vi "ANDOR_GetSoftwareVersion.vi"(7 "error in (no error)":errorcluster) -> (18 "Software Versions":T1, 20 "eprom":u32, 21 "cofFile":u32, 22 "vxdRev":u32, 23 "vxdVer":u32, 24 "dllRev":u32, 25 "dllVer":u32, 26 "DLL error code":u32, 27 "error out":errorcluster)   [LabVIEW 2010]
doc: "This function returns the Software version information for the microprocessor code and the driver.\n\n<B>Parameters:</B>\neprom - EPROM version\ncofFile - COF file version\nvxdRev - Driver revision number\nvxdVer - Driver version number\ndllRev - DLL revision number\ndllVer - DLL version number\n\n<B>Error codes:</B>\nDRV_SUCCESS - Version information returned.\nDRV_NOT_INITIALIZED - System not initialized.\nDRV_ACQUIRING - Acquisition in progress.\nDRV_ERROR_ACK - Unable to communicate with card."
uses:
  Program Files/Andor SOLIS/atmcd32d.dll
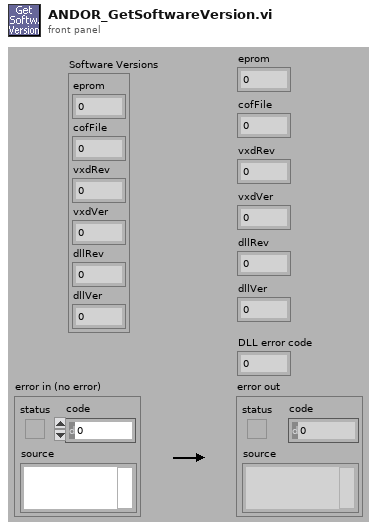
[diagram p1: front panel]
types:
  T1 = cluster{"eprom":u32, "cofFile":u32, "vxdRev":u32, "vxdVer":u32, "dllRev":u32, "dllVer":u32}
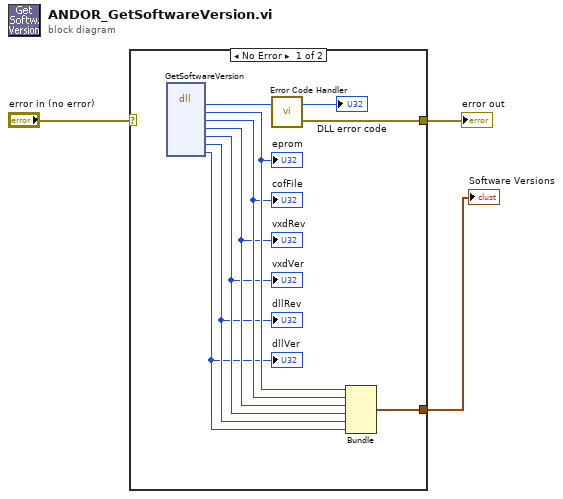
[diagram p0: block diagram]
diagram:
  n1 = case shown="No Error" "error in (no error)" {
    selector: "error in (no error)" -> [_ w14]
    tunnel: [w12 w14] -> w2
    tunnel: [w4 _] -> w1
    frame No Error {
      n2 = dll-call lib="C:/Program Files/Andor SOLIS/atmcd32d.dll" fn="GetSoftwareVersion"() -> ("return type"=w13:u32, "eprom"=w10:u32, "cofFile"=w9:u32, "vxdRev"=w8:u32, "vxdVer"=w7:u32, "dllRev"=w6:u32, "dllVer"=w5:u32)  [unwired: 9 in, 2 out]
      "eprom" <- w10
      "cofFile" <- w9
      "vxdRev" <- w8
      "vxdVer" <- w7
      "dllRev" <- w6
      "dllVer" <- w5
      n3 = call <userlib>:"Error Code Handler.vi"("DLL error code"=w13) -> ("error out"=w12:errorcluster, "dup DLL error code"=→"DLL error code":u32)  [unwired: 1 in]
      n4 = Bundle("eprom"=w10, "cofFile"=w9, "vxdRev"=w8, "vxdVer"=w7, "dllRev"=w6, "dllVer"=w5) -> (w4:T1)  [unwired: 1 in]
    }
    frame Error {
    }
  }
  "error out" <- w2
  "Software Versions" <- w1
